vi "Configure FIU Board.vi"(8 "error in (no error)":errorcluster, 10 "Slot #":T1 max=15, 11 "Rack #":u8) -> (0 "error out":errorcluster, 3 "SPI FIFO Messages":u64[](array[numeric]))   [LabVIEW 2014, in "SLSC configuration Shared.lvlib"]
doc: "Configures the DIO board (IOCON.BANK = 0 - sequential addressing, switch all pins to outputs)."
uses:
  CD/Source/Shared/SLSC configuration Shared.lvlib
  SPI Utility/Slot #.ctl
  CD/Source/Shared/Constants.vi
  MCP23S17/Update Mode All Pins.vi
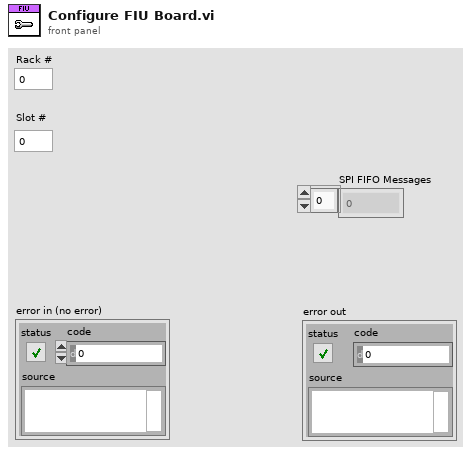
[diagram p1: front panel]
types:
  T1 = typedef "SLSC configuration Shared.lvlib/Slot #.ctl" = u8
  T2 = typedef "SLSC configuration Shared.lvlib/SPI Command.ctl" = cluster{"SPI Command":u32, "Transfer Length":u8}
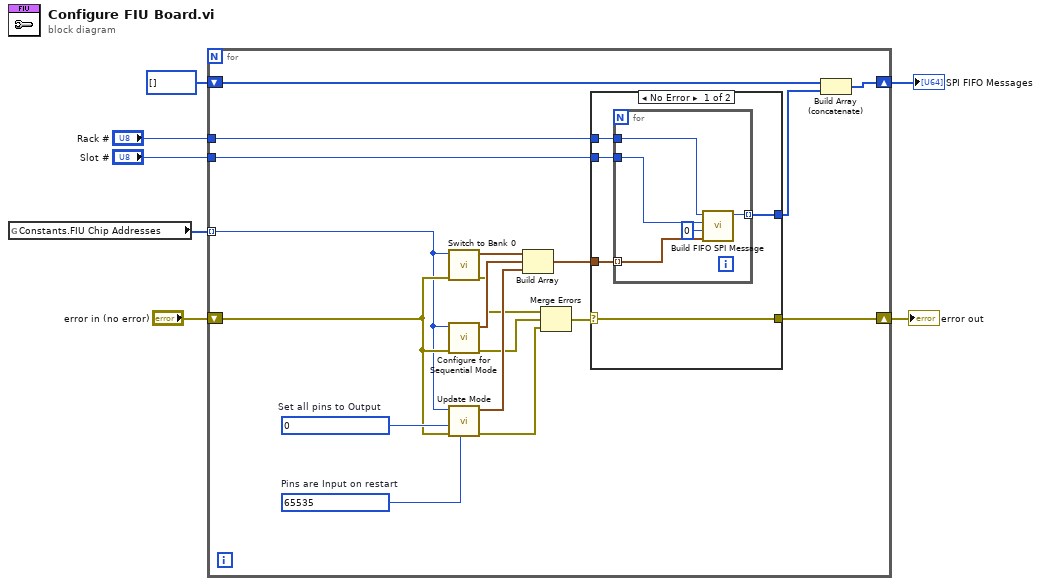
[diagram p0: block diagram]
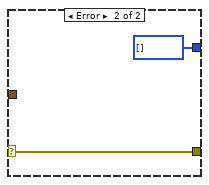
[diagram p2: hidden frame]
diagram:
  n1 = global read "Constants.vi" "Constants.FIU Chip Addresses"() -> (w1:u8[])
  n2 = for {
    tunnel: "Slot #" -> [w13]
    tunnel: "Rack #" -> [w12]
    shift-right: [w14] -> w5
    shift-left: "error in (no error)" -> [w23]
    tunnel: w1 -> [w11] mode=indexing
    shift-right: [w8] -> w6
    shift-left: u64[] [] -> [w10]
    w24 = u16 0  # Set all pins to Output
    w25 = u16 65535  # Pins are Input on restart
    n3 = call "Switch to Bank 0.vi"("error in (no error)"=w23, "Chip Address (A2 A1 A0)"=w11) -> ("error out"=w18:errorcluster, "SPI Command"=w22:T2)  [unwired: 8 in]
    n4 = call "Configure for Sequential Mode.vi"("error in (no error)"=w23, "Chip Address (A2 A1 A0)"=w11) -> ("error out"=w17:errorcluster, "SPI Command"=w21:T2)  [unwired: 8 in]
    n5 = call-poly "Update Mode.vi"("Mode Cache in"=w25, "error in (no error)"=w23, "Mode"=w24, "Chip Address (A2 A1 A0)"=w11) -> ("error out"=w16:errorcluster, "SPI Command"=w20:T2)  [unwired: 5 in, 1 out]
    n6 = Build Array(w22, w21, w20) -> (w19:T2[])
    n7 = Merge Errors(w18, w17, w16) -> (w15:errorcluster)
    n8 = case shown="No Error" w15 {
      selector: w15 -> [w28 w36]
      tunnel: w19 -> [w30 _]
      tunnel: [w29 u64[] []] -> w9
      tunnel: [w28 w36] -> w14
      tunnel: w13 -> [w27 _]
      tunnel: w12 -> [w26 _]
      frame No Error {
        n9 = for {
          tunnel: w30 -> [w34] mode=indexing
          tunnel: [w35] -> w29 mode=indexing
          tunnel: w27 -> [w33]
          tunnel: w26 -> [w32]
          n10 = call "Build FIFO SPI Message.vi"("SPI Command"=w34, "Chip Select"=u8 0, "Slot #"=w33, "Rack #"=w32) -> ("FIFO SPI Message"=w35:u64)  [unwired: 7 in]
        }
      }
      frame Error {
      }
    }
    n11 = Build Array (concatenate)(w10, w9) -> (w8:u64[])
  }
  "SPI FIFO Messages" <- w6
  "error out" <- w5
